vi "Untitled 1.vi"() -> ()   [LabVIEW 2019]
uses:
  <vilib>/picture/picture.llb/Draw 8-Bit Pixmap.vi
  F:/INO340/OSL/FITSdemo/fits/lib/testfits.dll
panel:
  out "FITS file image":picture
  in  "path":path
  out "Error message":string
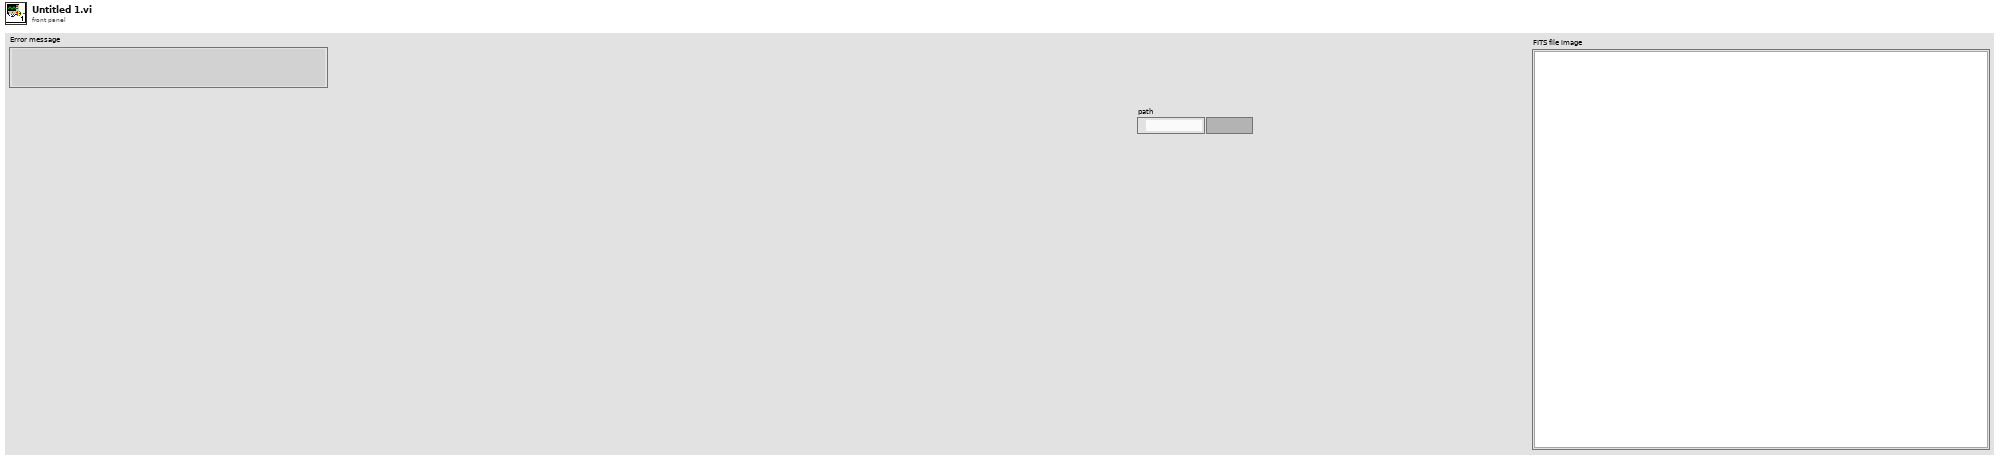
[diagram p1: front panel]
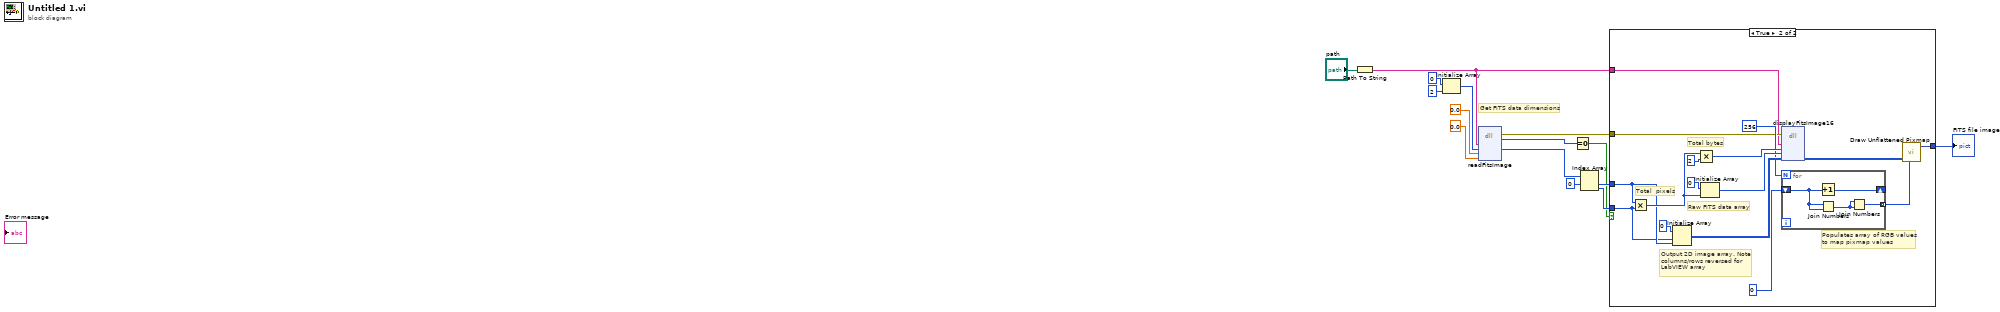
[diagram p0: block diagram]
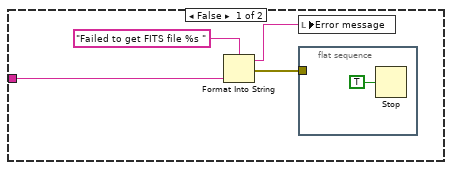
[diagram p2: hidden frame]
diagram:
  # "Get FITS data dimensions"
  n1 = Path To String(path="path") -> (string=w15:string)
  n2 = Initialize Array(0 ("element"), 2 ("dimension size")) -> (w11:i32[])
  n3 = dll-call lib="F:/INO340/OSL/FITSdemo/fits/lib/testfits.dll" fn="readFitsImage"("filename"=w15, "npix"=w11, "dmin"=sgl 0.0, "dmax"=sgl 0.0) -> (error out=w4:errorcluster, "return type"=w2:i32, "npix"=w8:i32[])  [unwired: 6 in, 1 out]
  n4 = Equal To 0?(x=w2) -> (x = 0?=w3:bool)
  n5 = Index Array(array=w8, index #1=0 ("index")) -> (element #1=w6:i32, element #2=w5:i32)  [unwired: 1 in]
  n6 = case shown="True" w3 {
    tunnel: w6 -> [_ w25]
    tunnel: w5 -> [_ w24]
    tunnel: w4 -> [_ w23]
    tunnel: w15 -> [w16 w22]
    tunnel: [_ w21] -> w1
    frame False {
      n7 = Format Into String(format string="Failed to get FITS file %s ", w16) -> (resulting string=w17:string, error out=w18:errorcluster)  [unwired: 2 in]
      n8 = local write "Error message"(w17) -> ()
      n9 = flat-sequence {
        tunnel: w18 -> [_]
        frame #0 {
          n10 = Stop(stop? (T)=TRUE) -> ()
        }
      }
    }
    frame True {
      # "Raw FITS data array"
      # "Output 2D image array. Note\ncolumns/rows reversed for\nLabVIEW array"
      # "Total bytes"
      # "Populates array of RGB values\nto map pixmap values"
      # "Total  pixels"
      n11 = Multiply(x=w25, y=w24) -> (x*y=w30:i32)
      n12 = Initialize Array(u8 0 ("element"), w24, w25) -> (w31:u8[][])
      n13 = Multiply(x=w30, y=2 ("Bytes per pixel")) -> (x*y=w34:i32)
      n14 = Initialize Array(i16 0 ("element"), w30) -> (w35:i16[])
      n15 = dll-call lib="F:/INO340/OSL/FITSdemo/fits/lib/testfits.dll" fn="displayFitsImage16"(error in=w23, "filename"=w22, "isize"=w34, "img"=w35, "outdat"=w31) -> ("outdat"=w26:u8[][])  [unwired: 6 in, 2 out]
      n16 = for {
        N: 256 -> [_]
        tunnel: [w40] -> w27 mode=indexing
        shift-right: [w39] -> _
        shift-left: u8 0 -> [w37]
        n17 = Increment(x=w37) -> (x+1=w39:u8)
        n18 = Join Numbers(hi=w37, lo=w37) -> ((hi.lo)=w38:u16)
        n19 = Join Numbers(hi=w38, lo=w38) -> ((hi.lo)=w40:u32)
      }
      n20 = call-poly <vilib>:"Draw Unflattened Pixmap.vi"("data"=w26, "color table"=w27) -> ("new picture"=w21:picture)  [unwired: 7 in]
    }
  }
  "FITS file image" <- w1
